vi "Configure Character Parameter.vi"(6 "value":u8, 7 "process number":u8, 8 "error in (no error)":errorcluster, 9 "parameter number":u8, 10 "node":u8, 11 "ProPar in":refnum<class "PL Bronkhorst ProPar.lvclass">) -> (0 "error out":errorcluster, 3 "ProPar out":refnum<class "PL Bronkhorst ProPar.lvclass">)   [LabVIEW 2015, in "PL Bronkhorst ProPar.lvclass"]
doc: "Configures specified character <b>parameter</b> of the specified <b>node</b>."
uses:
  PL Bronkhorst ProPar.lvclass
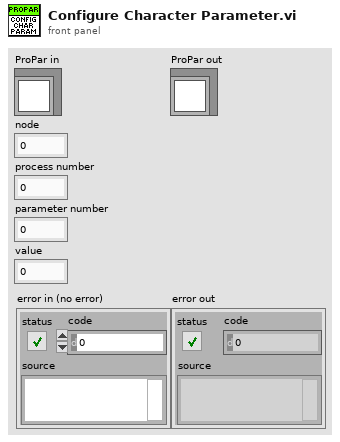
[diagram p1: front panel]
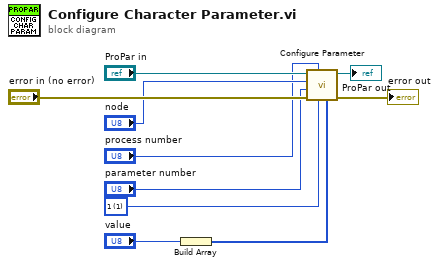
[diagram p0: block diagram]
diagram:
  w1 = u8 1 items=["variable"=0, "1"=1, "2"=2, "4"=4] ("value byte count")
  n1 = Build Array("value") -> (w2:u8[])
  n2 = call "Configure Parameter.vi"("value"=w2, "value byte count"=w1, "process number"="process number", "error in (no error)"="error in (no error)", "parameter number"="parameter number", "node"="node", "ProPar in"="ProPar in") -> ("error out"=→"error out":errorcluster, "ProPar out"=→"ProPar out":refnum<class "PL Bronkhorst ProPar.lvclass">)  [unwired: 3 in]
